vi "set_gate_parameters.vi"(4 "repetition period":dbl[unit], 5 "offset":dbl[unit], 6 "number of repetitions":i64, 7 "clock index":i32, 8 "error in (no error)":errorcluster, 9 "pulsing frequency":dbl[unit], 10 "number of pulses":i64, 11 "FPGAWrapperDL090211Galvo_grabber in":refnum<class "FPGAWrapperMM140723Galvo.lvclass">) -> (0 "error out":errorcluster, 3 "FPGAWrapperDL090211Galvo_grabber out":refnum<class "FPGAWrapperMM140723Galvo.lvclass">)   [LabVIEW 2010, in "FPGAWrapperMM140723Galvo.lvclass"]
doc: "Sets the timing parameters for the FPGA.\nclock index: which clock to set\noffset duration: delay until start of first train after \"start\" is issued\nhigh phase duration: duration, in which the gate is high (train of pulses)\nlow phase duration: output of pulses is supressed (pause)\npulse duration: period of the pulses (50% duty cycle)\nrepetitions: number of trains to issue"
uses:
  FPGAWrapperMM140723Galvo.lvclass
  type definitions/gate_cluster.ctl
  common_typedefs/gate_parameters_cluster.ctl
  FPGAWrapperMM140723Galvo.lvclass/FPGAWrapperMM140723Galvo.ctl
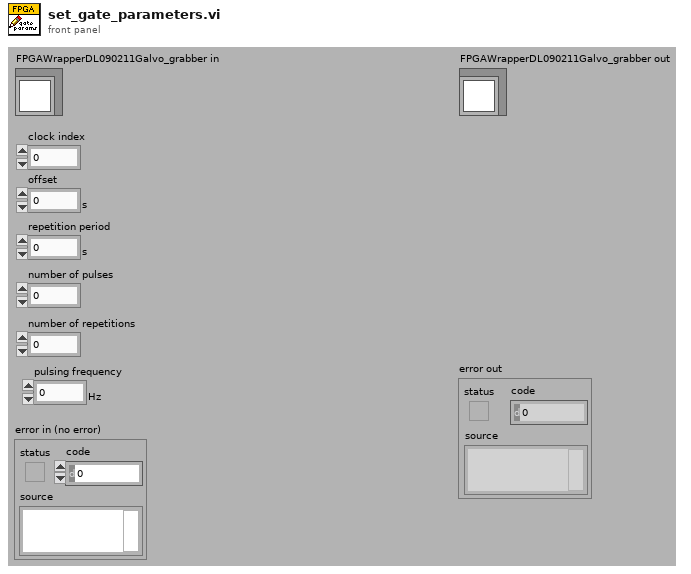
[diagram p1: front panel]
types:
  T1 = typedef "gate_cluster.ctl" = cluster{"index":i32, "parameters":T2}
  T2 = typedef "gate_parameters_cluster.ctl" = cluster{"offset":i64, "pulsing":i64, "not pulsing":i64, "cycles per pulse":i64, "repetitions":i64}
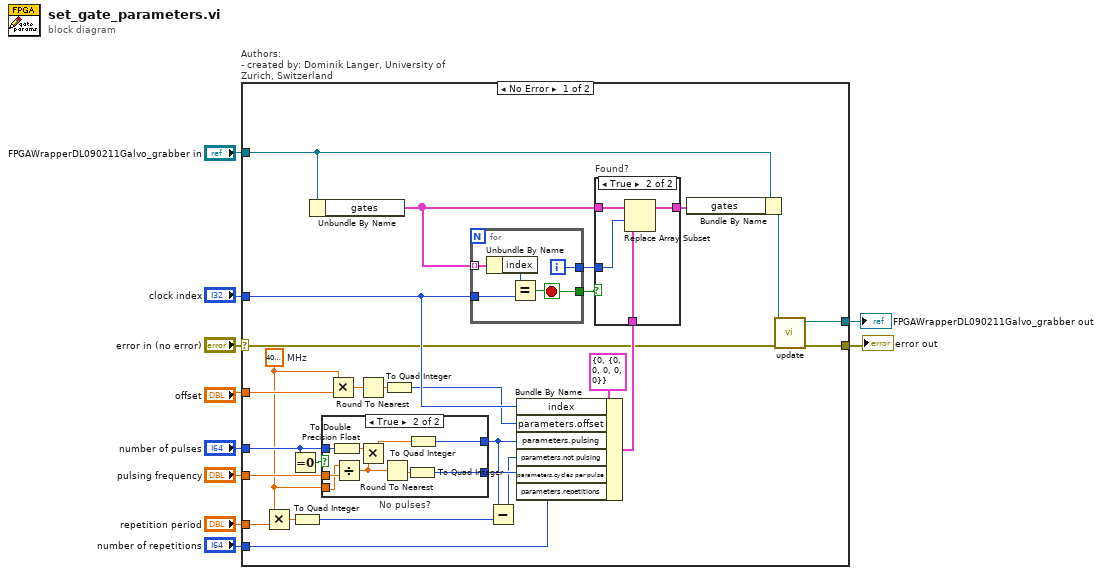
[diagram p0: block diagram]
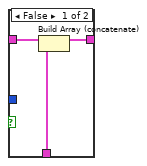
[diagram p3: hidden frame]
diagram:
  n1 = case "Authors: \n- created by: Dominik Langer, University of Zurich, Switzerland" shown="No Error" "error in (no error)" {
    selector: "error in (no error)" -> [w29 w59]
    tunnel: "FPGAWrapperDL090211Galvo_grabber in" -> [w36 w60]
    tunnel: [w26 w60] -> w9
    tunnel: [w28 w59] -> w8
    tunnel: "clock index" -> [w35 _]
    tunnel: "offset" -> [w25 _]
    tunnel: "number of repetitions" -> [w21 _]
    tunnel: "pulsing frequency" -> [w19 _]
    tunnel: "number of pulses" -> [w18 _]
    tunnel: "repetition period" -> [w15 _]
    frame No Error {
      w16 = dbl[unit] 40000000.0  # MHz
      n2 = Multiply(x=w16, y=w15) -> (x*y=w14:dbl)
      n3 = Equal To 0?(x=w18) -> (x = 0?=w17:bool)
      n4 = To Quad Integer(1:w14) -> (0:w12:i64)
      n5 = Unbundle By Name(w36) -> ("gates"=w34:T1[])
      n6 = case "No pulses?" shown="True" w17 {
        tunnel: [_ w46] -> w20
        tunnel: w19 -> [_ w44]
        tunnel: w16 -> [_ w38]
        tunnel: [_ w40] -> w13
        tunnel: w18 -> [_ w39]
        frame False {
        }
        frame True {
          n7 = To Double Precision Float(number=w39) -> (double precision float=w42:dbl)
          n8 = Divide(x=w38, y=w44) -> (x/y=w43:dbl)
          n9 = Multiply(x=w42, y=w43) -> (x*y=w41:dbl)
          n10 = Round To Nearest(number=w43) -> (nearest integer value=w45:dbl)
          n11 = To Quad Integer(1:w45) -> (0:w46:i64)
          n12 = To Quad Integer(1:w41) -> (0:w40:i64)
        }
      }
      n13 = Multiply(x=w16, y=w25) -> (x*y=w24:dbl)
      n14 = Round To Nearest(number=w24) -> (nearest integer value=w23:dbl)
      n15 = To Quad Integer(1:w23) -> (0:w22:i64)
      n16 = for {
        tunnel: w34 -> [w58] mode=indexing
        tunnel: w35 -> [w57]
        tunnel: [w55] -> w32
        tunnel: [w54] -> w30
        i -> [w55]
        stop <- w54 stop-if-true
        n17 = Unbundle By Name(w58) -> ("index"=w56:i32)
        n18 = Equal?(x=w56, y=w57) -> (x = y?=w54:bool)
      }
      n19 = Subtract(x=w13, y=w12) -> (x-y=w11:i64)
      n20 = Bundle By Name(cluster=T1 {"index"=0, "parameters"={"offset"=0, "pulsing"=0, "not pulsing"=0, "cycles per pulse"=0, "repetitions"=0}} ("gate"), "index"=w35, "parameters.offset"=w22, "parameters.pulsing"=w13, "parameters.not pulsing"=w11, "parameters.cycles per pulse"=w20, "parameters.repetitions"=w21) -> (w31:T1)
      n21 = case "Found?" shown="True" w30 {
        tunnel: w34 -> [w49 w53]
        tunnel: [w47 w52] -> w33
        tunnel: w32 -> [_ w51]
        tunnel: w31 -> [w48 w50]
        frame False {
          n22 = Build Array (concatenate)(w49, w48) -> (w47:T1[])
        }
        frame True {
          n23 = Replace Array Subset(array=w53, new element=w50, index=w51) -> (w52:T1[])
        }
      }
      n24 = Bundle By Name(cluster=w36, "gates"=w33) -> (w27:refnum<class "FPGAWrapperMM140723Galvo.lvclass">)
      n25 = call-dynamic "update.vi"("error in (no error)"=w29, "FPGAWrapperDL120115Galvo in"=w27) -> ("error out"=w28:errorcluster, "FPGAWrapperDL120115Galvo out"=w26:refnum<class "FPGAWrapperMM140723Galvo.lvclass">)  [unwired: 8 in]
    }
    frame Error {
    }
  }
  "error out" <- w8
  "FPGAWrapperDL090211Galvo_grabber out" <- w9
